vi "Create Write Endpoint.vi"(4 "Terminal":refnum<vi>, 6 "Type":T1, 8 "Index":i32, 9 "CBR Terminal":refnum<vi>, 10 "Close Tunnel":refnum<vi>, 11 "Write Frame":refnum<vi>) -> (0 "error out":errorcluster)   [LabVIEW 2020, in "FlexBlocks.lvlib"]
uses:
  FlexBlocks.lvlib
  Type Descriptor.ctl
  Terminal Direction.ctl
  Value Mode.ctl
  Special Terminal.ctl
  <vilib>/Utility/miscctls.llb/LVPointTypeDef.ctl
  Write Terminal Index.ctl
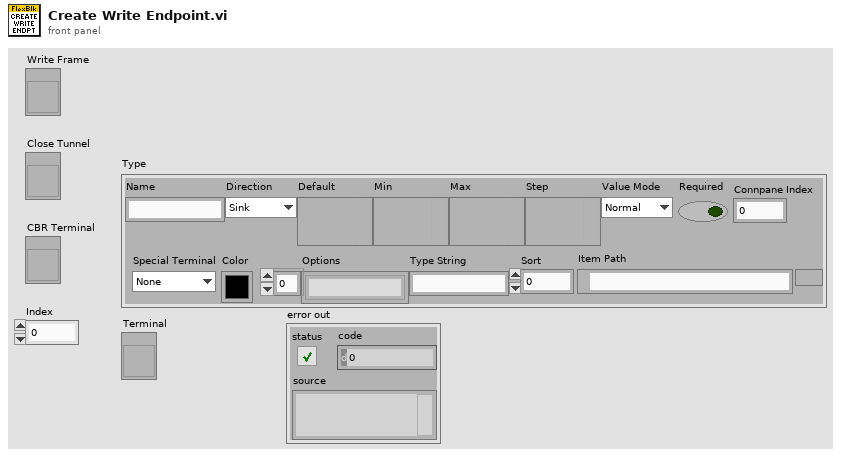
[diagram p1: front panel]
types:
  T1 = typedef "FlexBlocks.lvlib/Type Descriptor.ctl" = cluster{"Name":string, "Direction":T2, "Default":variant, "Min":variant, "Max":variant, "Step":variant, "Value Mode":T3, "Required":bool, "Connpane Index":i32, "Special Terminal":T4, "Color":u32, "Options":string[], "Type String":string, "Sort":i32, "Item Path":path}
  T2 = typedef "FlexBlocks.lvlib/Terminal Direction.ctl" = enum16{"Sink", "Source"}
  T3 = typedef "FlexBlocks.lvlib/Value Mode.ctl" = enum16{"Normal", "Range", "Select"}
  T4 = typedef "FlexBlocks.lvlib/Special Terminal.ctl" = enum16{"None", "Action", "Init", "Tag", "State in", "State out", "Error"}
  T5 = typedef "FlexBlocks.lvlib/Write Terminal Index.ctl" = enum16{"Timeout mS", "Timed Out", "Value", "Close", "Closed", "N/A 5", "FlexChannel", "N/A 7"}
  T6 = typedef "LVPointTypeDef.ctl" = cluster{"Horizontal":i16, "Vertical":i16}
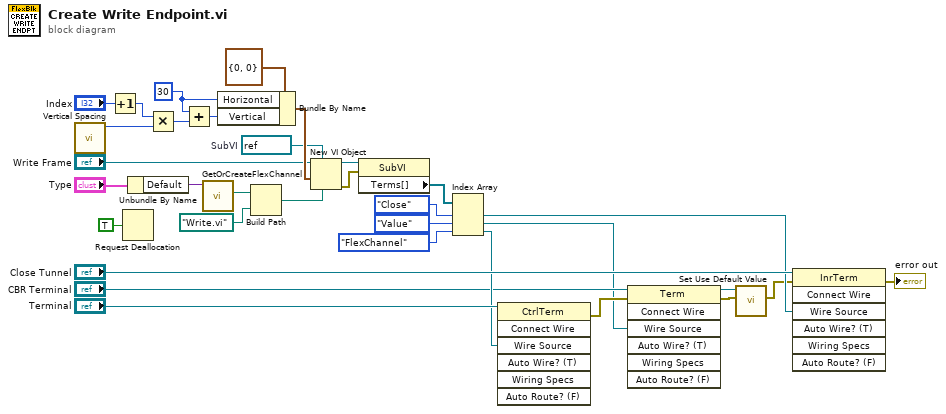
[diagram p0: block diagram]
diagram:
  w26 = 30 ("Left")
  w29 = refnum<vi> refnum  # SubVI
  n1 = call "Vertical Spacing.vi"() -> ("Spacing"=w32:i32)  [unwired: 11 in]
  n2 = Increment(x="Index") -> (x+1=w33:i32)
  n3 = Request Deallocation(TRUE ("flag")) -> ()
  n4 = Unbundle By Name("Type") -> ("Default"=w23:variant)
  n5 = Multiply(x=w33, y=w32) -> (x*y=w28:i32)
  n6 = Add(x=w26, y=w28) -> (x+y=w27:i32)
  n7 = call "GetOrCreateFlexChannel.vi"("Element Type"=w23) -> ("Channel Folder"=w21:path)  [unwired: 8 in, 2 out]
  n8 = Bundle By Name(cluster=T6 {"Horizontal"=0, "Vertical"=0} ("location"), "Horizontal"=w26, "Vertical"=w27) -> (w30:T6)
  n9 = Build Path(base path=w21, name or relative path=path "Write.vi") -> (appended path=w19:path)
  n10 = New VI Object(vi object class=w29, owner refnum="Write Frame", position/next to=w30, 6:w19) -> (object refnum=w17:refnum<vi>, 0:w16:errorcluster)  [unwired: 4 in]
  n11 = property class="SubVI"(reference=w17, error in=w16) -> ("Terms[]"=w15:refnum<vi>[])  [unwired: 2 out]
  n12 = Index Array(array=w15, index #1=Write_Terminal_Index."Close" ("Write Terminal Index"), index #2=Write_Terminal_Index."Value" ("Write Terminal Index"), index #3=Write_Terminal_Index."FlexChannel" ("Write Terminal Index")) -> (element #1=w10:refnum<vi>, element #2=w1:refnum<vi>, element #3=w7:refnum<vi>)
  n13 = invoke class="CtrlTerm" method="Connect Wire"(reference="Terminal", "Wire Source"=w7) -> (error out=w9:errorcluster)  [unwired: 5 in, 6 out]
  n14 = invoke class="Term" method="Connect Wire"(reference="CBR Terminal", error in=w9, "Wire Source"=w1) -> (reference out=w5:refnum<vi>, error out=w6:errorcluster)  [unwired: 4 in, 5 out]
  n15 = call "Set Use Default Value.vi"("error in (no error)"=w6, "Terminal"=w5) -> ("error out"=w4:errorcluster)  [unwired: 9 in]
  n16 = invoke class="InrTerm" method="Connect Wire"(reference="Close Tunnel", error in=w4, "Wire Source"=w10) -> (error out=→"error out":errorcluster)  [unwired: 4 in, 6 out]
